vi "Interpolation method for Hanning Win RT.vi"(8 "Prev Amp":dbl, 9 "Next Amp":dbl, 10 "Max Amp":dbl, 11 "Max Bin":i32) -> (3 "Bin":dbl)   [LabVIEW 2014]
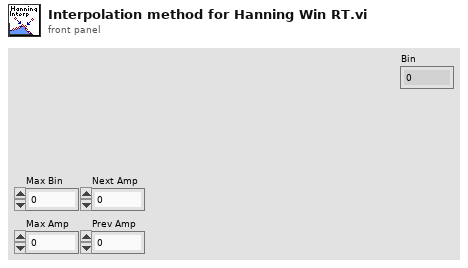
[diagram p1: front panel]
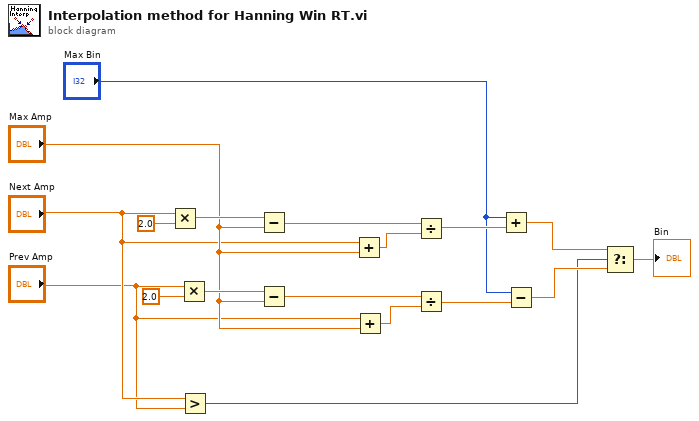
[diagram p0: block diagram]
diagram:
  n1 = Multiply(x="Next Amp", y=2.0) -> (x*y=w16:dbl)
  n2 = Multiply(x="Prev Amp", y=2.0) -> (x*y=w15:dbl)
  n3 = Greater?(x="Next Amp", y="Prev Amp") -> (0:w1:bool)
  n4 = Subtract(x=w16, y="Max Amp") -> (x-y=w14:dbl)
  n5 = Subtract(x=w15, y="Max Amp") -> (x-y=w13:dbl)
  n6 = Add(x="Next Amp", y="Max Amp") -> (x+y=w12:dbl)
  n7 = Add(x="Prev Amp", y="Max Amp") -> (x+y=w11:dbl)
  n8 = Divide(x=w14, y=w12) -> (x/y=w9:dbl)
  n9 = Divide(x=w13, y=w11) -> (x/y=w8:dbl)
  n10 = Add(x="Max Bin", y=w9) -> (x+y=w6:dbl)
  n11 = Subtract(x="Max Bin", y=w8) -> (x-y=w5:dbl)
  n12 = Select(t=w6, s=w1, f=w5) -> (s? t:f=→"Bin":dbl)
